vi "handle.vi"(5 "TCP connection":refnum<k5>, 7 "response queue":refnum<queue>, 9 "server information":T1, 10 "application request in":T2, 11 "http responder in":refnum<class "http responder.lvclass">) -> (0 "stop processing":bool, 3 "http responder out":refnum<class "http responder.lvclass">)   [LabVIEW 2016, in "http responder.lvclass"]
uses:
  http responder.lvclass
  HTTP server/http response.ctl
  HTTP server/http response packet type.ctl
  HTTP headers/http header data.ctl
  HTTP server/http request.ctl
  HTTP server/http method.ctl
  HTTP server/http server info.ctl
  HTTP server/Basic HTTP server.lvclass
  HTTP headers/http headers.lvlib
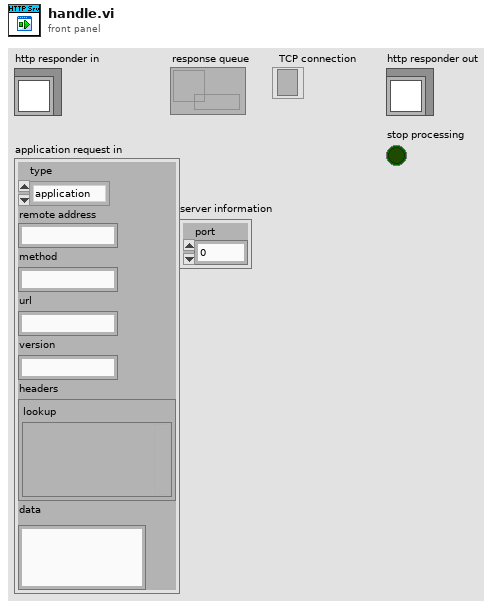
[diagram p1: front panel]
types:
  T1 = typedef "Basic HTTP server.lvclass/http server info.ctl" = cluster{"port":u16}
  T2 = typedef "Basic HTTP server.lvclass/http request.ctl" = cluster{"type":T3, "remote address":string, "method":string, "url":string, "version":string, "headers":T4, "data":string}
  T3 = typedef "Basic HTTP server.lvclass/http method.ctl" = enum16{"application", "error", "upgrade", "expect"}
  T4 = typedef "http headers.lvlib/http header data.ctl" = cluster{"lookup":variant}
  T5 = typedef "Basic HTTP server.lvclass/http response packet type.ctl" = enum16{"full response", "header only", "data only", "last data", "raw output"}
  T6 = typedef "Basic HTTP server.lvclass/http response.ctl" = cluster{"packet type":T5, "reason code":u16, "status string":string, "headers":T4, "cookies":string[], "data":string}
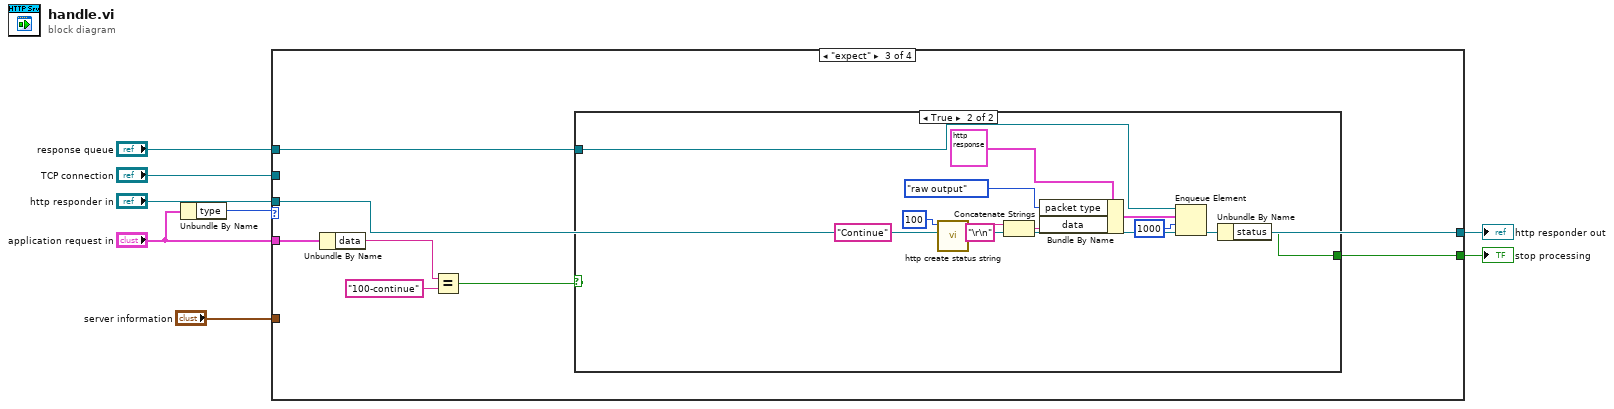
[diagram p0: block diagram]
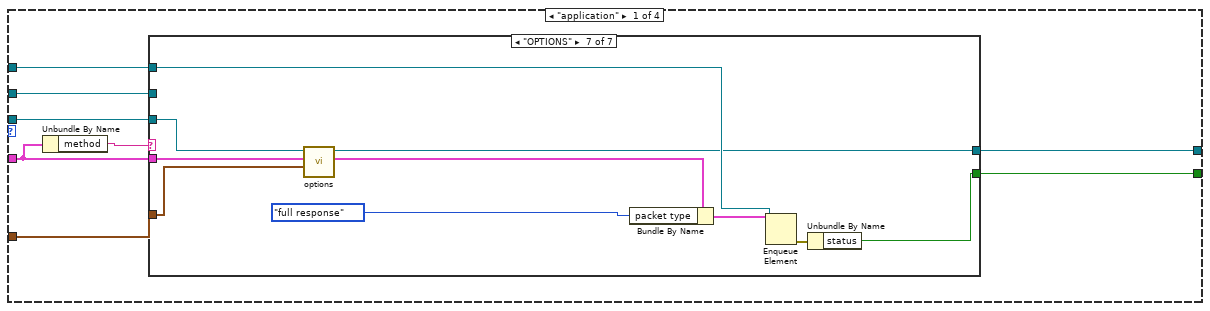
[diagram p2: hidden frame]
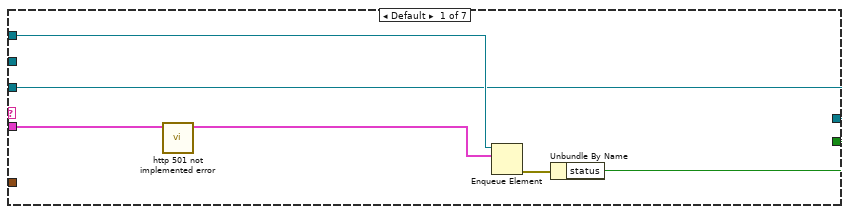
[diagram p3: hidden frame]
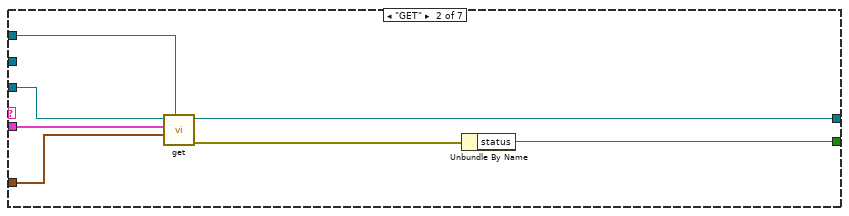
[diagram p4: hidden frame]
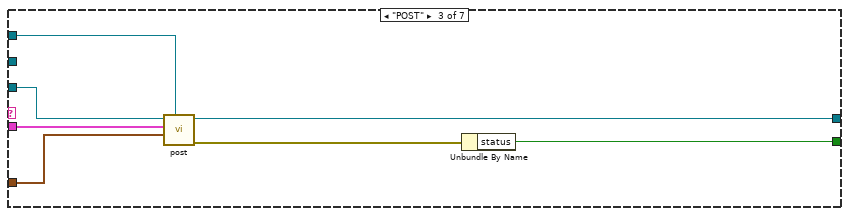
[diagram p5: hidden frame]
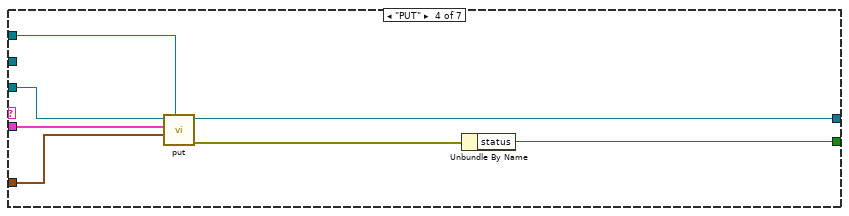
[diagram p6: hidden frame]
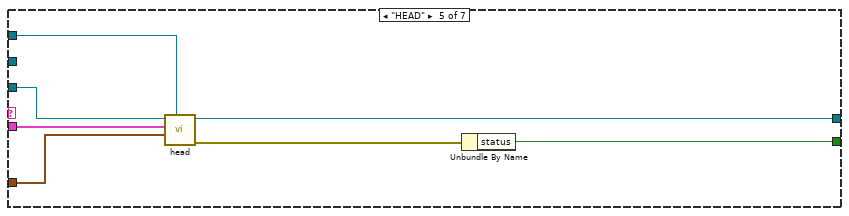
[diagram p7: hidden frame]
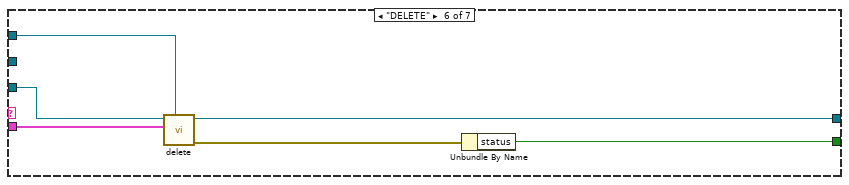
[diagram p8: hidden frame]
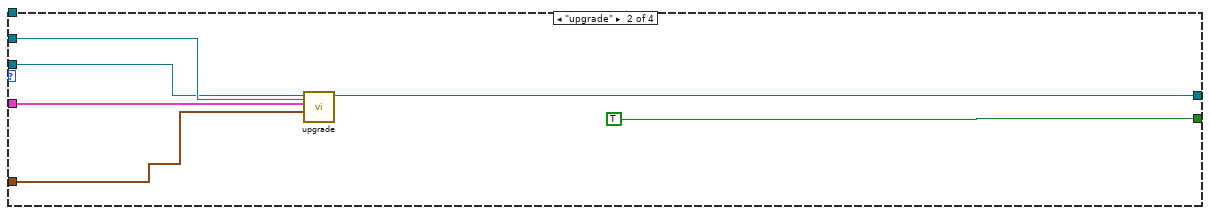
[diagram p9: hidden frame]
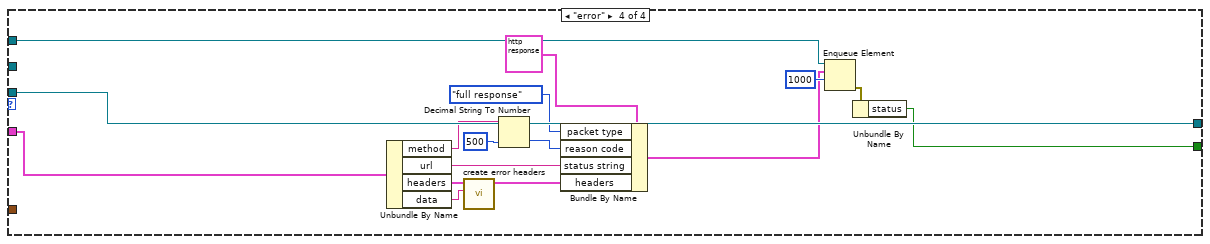
[diagram p11: hidden frame]
diagram:
  n1 = Unbundle By Name("application request in") -> ("type"=w1:T3)
  n2 = case shown="\"expect\"" w1 {
    tunnel: [w16 TRUE ("status") w73 w104] -> w8
    tunnel: "application request in" -> [w10 w71 w78 w107]
    tunnel: "TCP connection" -> [w15 w70 _ _]
    tunnel: "response queue" -> [w14 _ w75 w105]
    tunnel: "http responder in" -> [w13 w69 w77 w106]
    tunnel: [w12 w68 w77 w106] -> w3
    tunnel: "server information" -> [w11 w67 _ _]
    frame "application" {
      n3 = Unbundle By Name(w10) -> ("method"=w9:string)
      n4 = case shown="\"OPTIONS\"" w9 {
        tunnel: w10 -> [w22 w24 w31 w38 w45 w51 w59]
        tunnel: [w18 w29 w36 w43 w50 w56 w64] -> w16
        tunnel: w14 -> [w20 w25 w32 w39 w46 w52 w65]
        tunnel: w15 -> [_ _ _ _ _ _ _]
        tunnel: w13 -> [w17 w28 w35 w42 w49 w55 w61]
        tunnel: [w17 w27 w34 w41 w48 w54 w58] -> w12
        tunnel: w11 -> [_ w23 w30 w37 w44 _ w57]
        frame Default {
          n5 = call "http 501 not implemented error.vi"("application request in"=w22) -> ("application request out"=w19:T6)  [unwired: 10 in]
          n6 = Enqueue Element(queue=w20, element=w19) -> (error out=w21:errorcluster)  [unwired: 2 in, 2 out]
          n7 = Unbundle By Name(w21) -> ("status"=w18:bool)
        }
        frame "GET" {
          n8 = call-dynamic "get.vi"("transmit queue"=w25, "server information"=w23, "application request in"=w24, "http responder in"=w28) -> ("error out"=w26:errorcluster, "http responder out"=w27:refnum<class "http responder.lvclass">)  [unwired: 6 in]
          n9 = Unbundle By Name(w26) -> ("status"=w29:bool)
        }
        frame "POST" {
          n10 = call-dynamic "post.vi"("transmit queue"=w32, "server information"=w30, "application request in"=w31, "http responder in"=w35) -> ("error out"=w33:errorcluster, "http responder out"=w34:refnum<class "http responder.lvclass">)  [unwired: 6 in]
          n11 = Unbundle By Name(w33) -> ("status"=w36:bool)
        }
        frame "PUT" {
          n12 = call-dynamic "put.vi"("transmit queue"=w39, "server information"=w37, "application request in"=w38, "http responder in"=w42) -> ("error out"=w40:errorcluster, "http responder out"=w41:refnum<class "http responder.lvclass">)  [unwired: 6 in]
          n13 = Unbundle By Name(w40) -> ("status"=w43:bool)
        }
        frame "HEAD" {
          n14 = call-dynamic "head.vi"("transmit queue"=w46, "server information"=w44, "application request in"=w45, "http responder in"=w49) -> ("error out"=w47:errorcluster, "http responder out"=w48:refnum<class "http responder.lvclass">)  [unwired: 6 in]
          n15 = Unbundle By Name(w47) -> ("status"=w50:bool)
        }
        frame "DELETE" {
          n16 = call-dynamic "delete.vi"("transmit queue"=w52, "application request in"=w51, "http responder in"=w55) -> ("error out"=w53:errorcluster, "http responder out"=w54:refnum<class "http responder.lvclass">)  [unwired: 7 in]
          n17 = Unbundle By Name(w53) -> ("status"=w56:bool)
        }
        frame "OPTIONS" {
          n18 = call-dynamic "options.vi"("server information"=w57, "application request in"=w59, "http responder in"=w61) -> ("application response out"=w60:T6, "http responder out"=w58:refnum<class "http responder.lvclass">)  [unwired: 7 in]
          n19 = Bundle By Name(cluster=w60, "packet type"=http_response_packet_type."full response") -> (w63:T6)
          n20 = Enqueue Element(queue=w65, element=w63) -> (error out=w66:errorcluster)  [unwired: 2 in, 2 out]
          n21 = Unbundle By Name(w66) -> ("status"=w64:bool)
        }
      }
    }
    frame "upgrade" {
      n22 = call "upgrade.vi"("tcp conn"=w70, "server information"=w67, "application request in"=w71, "http responder in"=w69) -> ("http responder out"=w68:refnum<class "http responder.lvclass">)  [unwired: 7 in]
    }
    frame "expect" {
      n23 = Unbundle By Name(w78) -> ("data"=w76:string)
      n24 = Equal?(x=w76, y="100-continue") -> (x = y?=w74:bool)
      n25 = case shown="True" w74 {
        tunnel: w75 -> [_ w91]
        tunnel: [_ w82] -> w73
        frame False {
        }
        frame True {
          n26 = call "http create status string.vi"("status string"="Continue", "reason code"=u16 100) -> ("status line"=w85:string)  [unwired: 9 in]
          n27 = Concatenate Strings(w85, "\r\n" ("string")) -> (w81:string)
          n28 = Bundle By Name(cluster=T6 {"packet type"=enum."full response", "reason code"=0, "status string"="", "headers"={"lookup"=variant}, "cookies"=[], "data"=""} ("element"), "packet type"=http_response_packet_type."raw output", "data"=w81) -> (w89:T6)
          n29 = Enqueue Element(queue=w91, element=w89, timeout in ms (-1)=1000) -> (error out=w83:errorcluster)  [unwired: 1 in, 2 out]
          n30 = Unbundle By Name(w83) -> ("status"=w82:bool)
        }
      }
    }
    frame "error" {
      n31 = Unbundle By Name(w107) -> ("method"=w98:string, "url"=w93:string, "headers"=w95:T4, "data"=w92:string)
      n32 = call "create error headers.vi"("custom error reason"=w92, "headers in"=w95) -> ("headers out"=w94:T4)  [unwired: 9 in]
      n33 = Decimal String To Number(string=w98, default (0L)=500 ("default (0 I32)")) -> (number=w96:i32)  [unwired: 1 in, 1 out]
      n34 = Bundle By Name(cluster=T6 {"packet type"=enum."full response", "reason code"=0, "status string"="", "headers"={"lookup"=variant}, "cookies"=[], "data"=""} ("application request"), "packet type"=http_response_packet_type."full response", "reason code"=w96, "status string"=w93, "headers"=w94) -> (w99:T6)
      n35 = Enqueue Element(queue=w105, element=w99, timeout in ms (-1)=1000) -> (error out=w102:errorcluster)  [unwired: 1 in, 2 out]
      n36 = Unbundle By Name(w102) -> ("status"=w104:bool)
    }
  }
  "http responder out" <- w3
  "stop processing" <- w8
